vi "Capture the Project refs.vi"(8 "error in":errorcluster, 10 "Target Selection":string, 11 "Project Selection":string) -> (0 "error out":errorcluster, 3 "References":T1)   [LabVIEW 2019, in "Panther Dashboard.lvlib"]
uses:
  Panther Dashboard.lvlib
  Project References--cluster.ctl
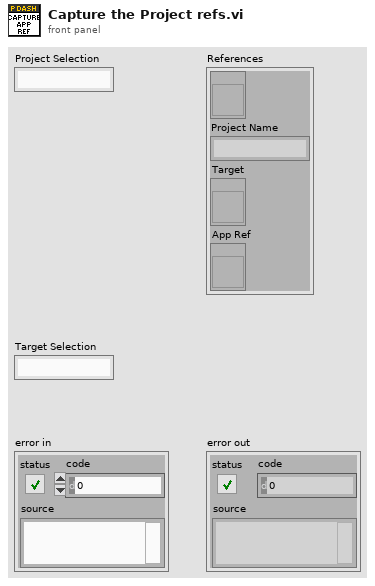
[diagram p1: front panel]
types:
  T1 = typedef "Panther Dashboard.lvlib/Project References--cluster.ctl" = cluster{"Project Ref":refnum<vi>, "Project Name":string, "Target":refnum<vi>, "App Ref":refnum<vi>}
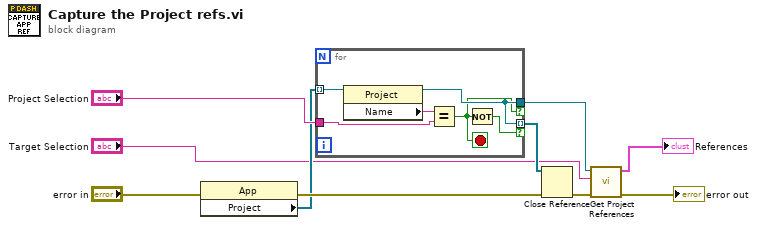
[diagram p0: block diagram]
diagram:
  n1 = property class="App"(error in="error in") -> (error out=w8:errorcluster, "Project"=w3:refnum<vi>[])  [unwired: 1 in, 1 out]
  n2 = for {
    tunnel: w3 -> [w16] mode=indexing
    tunnel: [w13] -> w5 if=w12
    tunnel: "Project Selection" -> [w14]
    tunnel: [w13] -> w2 mode=indexing if=w11
    stop <- w12 stop-if-true
    n3 = property class="Project"(reference=w16) -> (reference out=w13:refnum<vi>, "Name"=w15:string)  [unwired: 1 in, 1 out]
    n4 = Equal?(x=w15, y=w14) -> (x = y?=w12:bool)
    n5 = Not(x=w12) -> (.not. x?=w11:bool)
  }
  n6 = Close Reference(reference=w2, error in (no error)=w8) -> (error out=w7:errorcluster)
  n7 = call "Get Project References.vi"("error in"=w7, "Target Selection"="Target Selection", "Project in"=w5) -> ("error out"=→"error out":errorcluster, "References"=→"References":T1)  [unwired: 7 in]
